vi "Teleop.vi"(10 "Match Info":T1={"Autonomous Elapsed Seconds"=0.0, "TeleOp Elapsed Seconds"=0.0, "Disabled Elapsed Seconds"=0.0, "Visited Autonomous"=FALSE, "Visited TeleOp"=FALSE, "Visited Disabled"=FALSE, "Autonomous Settings"={"Autonomous Style"=enum."Independent", "VI Refnum"=refnum}}, 11 "Call Context":T2) -> ()   [LabVIEW 2018]
doc: "This VI is called for each TeleOp packet received from the DS where the robot is not disabled. It is often used to read from the joysticks and update I/O or to update setpoints for timed control loops. It should complete and return within 20 milliseconds or it may miss DS packets."
uses:
  <vilib>/Rock Robotics/WPI/DriverStation/WPI_DriverStationDerivedRobotMode.ctl
  <vilib>/Rock Robotics/WPI/DriverStation/WPI_DriverStationMatch Info.ctl
  <vilib>/Rock Robotics/WPI/ThirdParty/Phoenix-LabVIEW/Motor Controller/Controls/CTRE_Phoenix_MotorControl_ControlMode.ctl
  <vilib>/Rock Robotics/Network Tables/NT Read Boolean.vi
  <vilib>/Rock Robotics/Network Tables/NT Read Number.vi
  <vilib>/Rock Robotics/WPI/Utilities/WPI_GetSetVariantRefNum.vi
  <vilib>/Rock Robotics/Network Tables/NT Write Boolean Array.vi
  <vilib>/Rock Robotics/Network Tables/NT Write Numeric Array.vi
  <vilib>/Rock Robotics/WPI/ThirdParty/Phoenix-LabVIEW/Motor Controller/Get/CTRE_Phoenix_MotorController_GetSelectedSensorData.vi
panel:
  out "Angle Back Left":dbl
  out "Angle Back Right":dbl
  out "Angle Front Right":dbl
  out "Angle Front Left":dbl
  out "Speed Back Left":dbl
  out "Speed Back Right":dbl
  out "Speed Front Right":dbl
  out "Speed Front Left":dbl
  in  "reverse steer":bool=TRUE
  in  "reverse encoder":bool=TRUE
  in  "ScaleSpeed":dbl=1.0
  in  "upper limit":dbl=0.02
  in  "lower limit":dbl=-0.02
  in  "Wheelbase":dbl=23.75
  in  "Trackwidth":dbl=18.1
  out "Sample Slider 0":dbl(slide) scale=0.0..5.0
  out "Sample Boolean 1":bool
  out "Sample Boolean 0":bool
  # "This column has configuration\nconstants for the swerve\ndrives. ReverseSteer and \nRevereEncoder should stay\n\"on\" (true) unless your hardware\nrequires it to be set otherwise."
  # "This column is debug \noutput for the 4 swerve\ndrives - wheel speed and \nangle info."
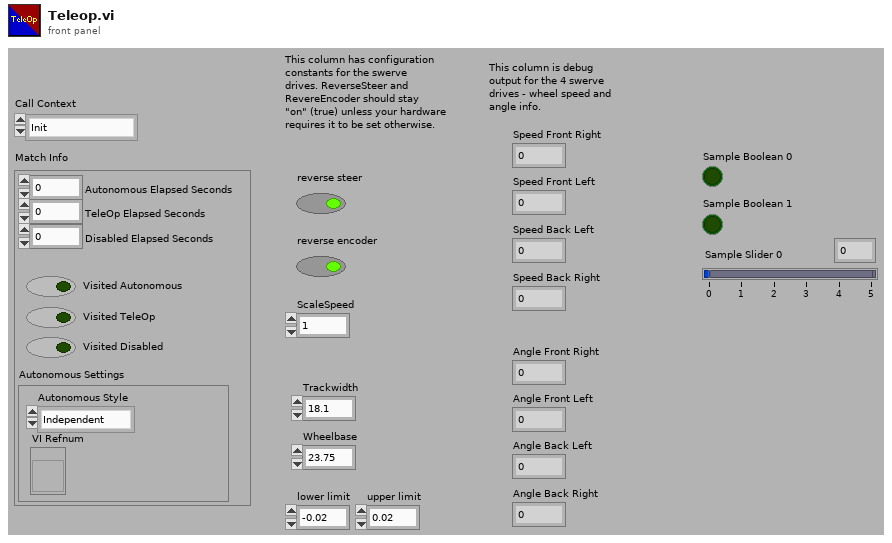
[diagram p1: front panel]
types:
  T1 = typedef "WPI_DriverStationMatch Info.ctl" = cluster{"Autonomous Elapsed Seconds":dbl, "TeleOp Elapsed Seconds":dbl, "Disabled Elapsed Seconds":dbl, "Visited Autonomous":bool, "Visited TeleOp":bool, "Visited Disabled":bool, "Autonomous Settings":cluster{"Autonomous Style":enum16{"Iterative", "Independent"}, "VI Refnum":refnum<vi>}}
  T2 = typedef "WPI_DriverStationDerivedRobotMode.ctl" = enum16{"Init", "Execute", "Stop"}
  T3 = typedef "CTRE_Phoenix_MotorControl_ControlMode.ctl" = u16
  T4 = typedef "WPI_JoystickDevRef.ctl" = cluster{"Device":T5}
  T5 = typedef "WPI_JoystickDeviceEnum.ctl" = enum16{"USB 0", "USB 1", "USB 2", "USB 3", "USB 4", "USB 5"}
  T6 = typedef "WPI_MotorControlDeviceRef.ctl" = cluster{"DeviceStatus":errorcluster, "Type":T7, "PWM":cluster{"PWM Channel":T8, "DeadBand":T9}, "CAN":cluster{"Device Number":u8, "SetOutput VI Ref":variant, "GetOutput VI Ref":variant, "Enable VI Ref":variant, "Disable VI Ref":variant, "Data":variant}, "Invert":bool, "DIO PWM":cluster{"PWM \"Enable\" Channel":T8, "DIOChannel":T10, "PWM Rate":dbl}}
  T7 = typedef "WPI_MotorControlType.ctl" = enum16{"PWM", "CAN", "DIO PWM"}
  T8 = typedef "FPGA_DIOPWMChannel.ctl" = enum8{"PWM 0", "PWM 1", "PWM 2", "PWM 3", "PWM 4", "PWM 5", "PWM 6", "PWM 7", "PWM 8", "PWM 9", "PWM MXP 0", "PWM MXP 1", "PWM MXP 2", "PWM MXP 3", "PWM MXP 4", "PWM MXP 5", "PWM MXP 6", "PWM MXP 7", "PWM MXP 8", "PWM MXP 9", "Invalid"}
  T9 = typedef "WPI_PWMDeadband.ctl" = cluster{"Name":string, "maxPositivePwm":i32, "minPositivePwm":i32, "centerPwm":i32, "maxNegativePwm":i32, "minNegativePwm":i32, "angularRange":u16}
  T10 = typedef "FPGA_DIOChannel.ctl" = enum8{"DIO 0", "DIO 1", "DIO 2", "DIO 3", "DIO 4", "DIO 5", "DIO 6", "DIO 7", "DIO 8", "DIO 9", "DIO MXP 0", "DIO MXP 1", "DIO MXP 2", "DIO MXP 3", "DIO MXP 4", "DIO MXP 5", "DIO MXP 6", "DIO MXP 7", "DIO MXP 8", "DIO MXP 9", "DIO MXP 10", "DIO MXP 11", "DIO MXP 12", "DIO MXP 13", "DIO MXP 14", "DIO MXP 15", "SPI Port CS1", "SPI Port CS2", "SPI Port CS3", "SPI Port MISO", "SPI Port MOSI", "Invalid"}
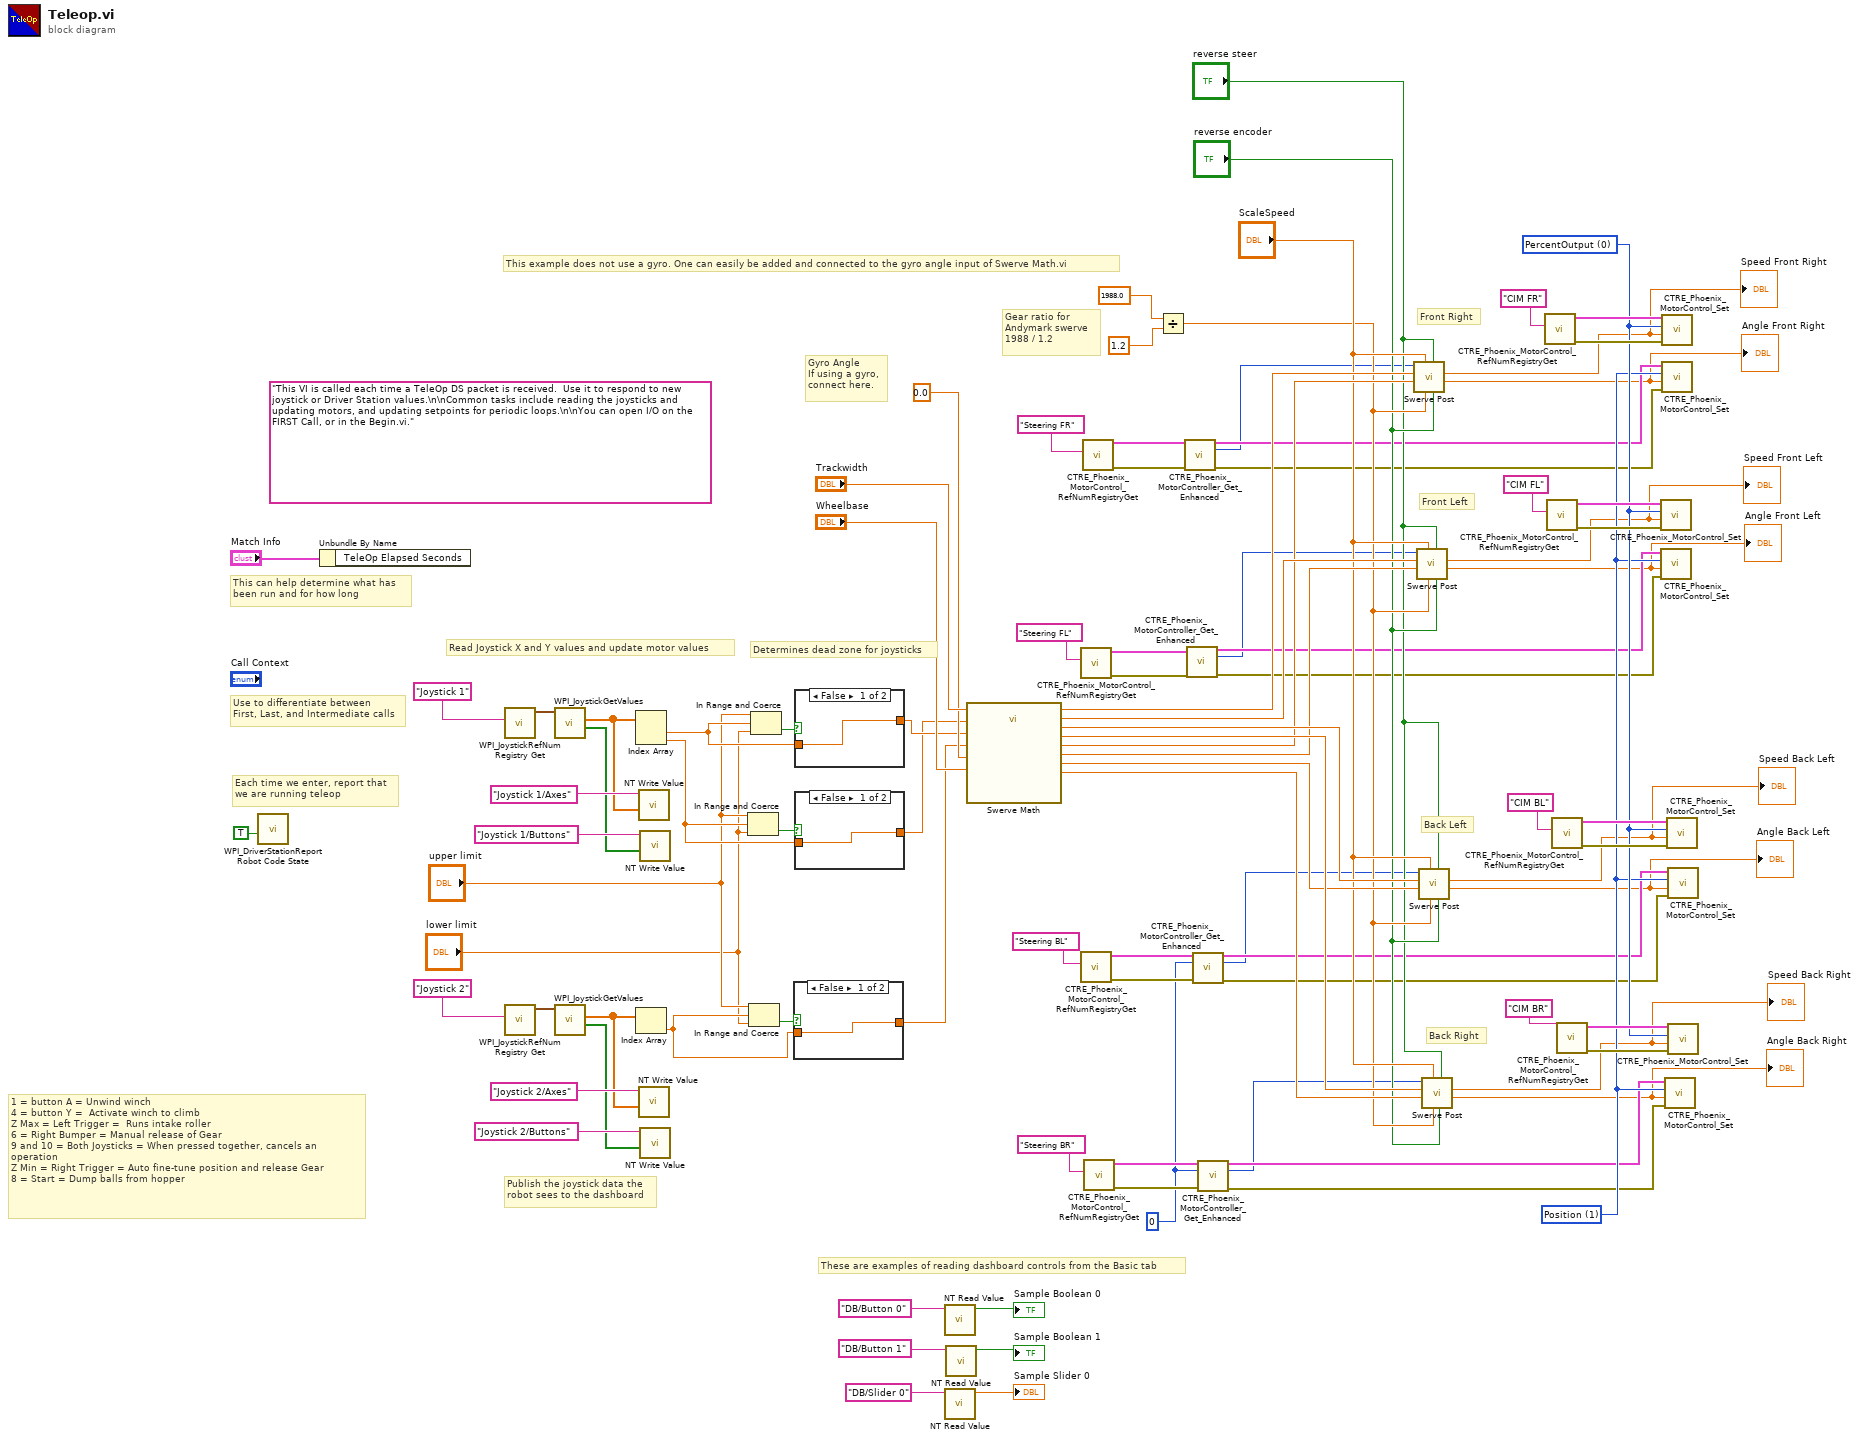
[diagram p0: block diagram]
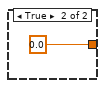
[diagram p2: hidden frame]
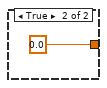
[diagram p3: hidden frame]
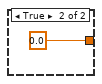
[diagram p4: hidden frame]
diagram:
  w22 = u32 0 ("pidLoopIdx")
  w31 = T3 1 items=["PercentOutput"=0, "Position"=1, "Velocity"=2, "Current"=3, "Follower"=5, "MotionProfile"=6, "MotionMagic"=7, "MotionProfileArc"=10, "Disabled"=15] ("Control Mode")
  w32 = T3 0 items=["PercentOutput"=0, "Position"=1, "Velocity"=2, "Current"=3, "Follower"=5, "MotionProfile"=6, "MotionMagic"=7, "MotionProfileArc"=10, "Disabled"=15] ("Control Mode")
  (unwired) "This VI is called each time a TeleOp DS packet is received.  Use it to respond to new joystick or Driver Station values.\n\nCommon tasks include reading the joysticks and updating motors, and updating setpoints for periodic loops.\n\nYou can open I/O on the FIRST Call, or in the Begin.vi."
  # "Gear ratio for\nAndymark swerve\n1988 / 1.2"
  # "Back Right"
  # "Back Left"
  # "Front Left"
  # "Front Right"
  # "This example does not use a gyro. One can easily be added and connected to the gyro angle input of Swerve Math.vi"
  # "1 = button A =\tUnwind winch\n4 = button Y = \tActivate winch to climb\nZ Max = Left Trigger = \tRuns intake roller\n6 = Right Bumper = Manual release of Gear\n9 and 10 = Both Joysticks = When pressed together, cancels an operation\nZ Min = Right Trigger = Auto fine-tune position and release Gear \n8 = Start = Dump balls from hopper"
  # "Determines dead zone for joysticks"
  # "Gyro Angle\nIf using a gyro,\nconnect here."
  # "Publish the joystick data the\nrobot sees to the dashboard"
  # "These are examples of reading dashboard controls from the Basic tab"
  # "Each time we enter, report that\nwe are running teleop"
  # "Use to differentiate between\nFirst, Last, and Intermediate calls"
  # "This can help determine what has\nbeen run and for how long"
  # "Read Joystick X and Y values and update motor values"
  n1 = call <vilib>:"WPI_DriverStationReport Robot Code State.vi"("TeleOp"=TRUE ("Autonomous")) -> ()  [unwired: 10 in, 1 out]
  n2 = Unbundle By Name("Match Info") -> ()  [unwired: 1 out]
  n3 = call <vilib>:"WPI_JoystickRefNum Registry Get.vi"("refnum name"="Joystick 1") -> ("JoystickDevRef"=w86:T4)  [unwired: 1 in, 9 out]
  n4 = call <vilib>:"WPI_JoystickRefNum Registry Get.vi"("refnum name"="Joystick 2") -> ("JoystickDevRef"=w80:T4)  [unwired: 1 in, 9 out]
  n5 = call <vilib>:"WPI_JoystickGetValues.vi"("JoystickDevRef"=w86) -> ("Buttons"=w82:bool[], "Axes"=w83:dbl[])  [unwired: 6 in, 3 out]
  n6 = call <vilib>:"WPI_JoystickGetValues.vi"("JoystickDevRef"=w80) -> ("Buttons"=w76:bool[], "Axes"=w77:dbl[])  [unwired: 6 in, 3 out]
  n7 = Index Array(array=w83) -> (element #1=w56:dbl, element #2=w58:dbl)  [unwired: 2 in]
  n8 = Index Array(array=w77) -> (element=w57:dbl)  [unwired: 1 in]
  n9 = call-poly <vilib>:"NT Write Value.vi"("Numeric Array"=w83, "Name"="Joystick 1/Axes") -> ()  [unwired: 9 in, 1 out]
  n10 = call-poly <vilib>:"NT Write Value.vi"("Numeric Array"=w77, "Name"="Joystick 2/Axes") -> ()  [unwired: 9 in, 1 out]
  n11 = call-poly <vilib>:"NT Write Value.vi"("Boolean Array"=w82, "Name"="Joystick 1/Buttons") -> ()  [unwired: 9 in, 1 out]
  n12 = call-poly <vilib>:"NT Write Value.vi"("Boolean Array"=w76, "Name"="Joystick 2/Buttons") -> ()  [unwired: 9 in, 1 out]
  n13 = In Range and Coerce(upper limit="upper limit", x=w58, lower limit="lower limit") -> (In Range?=w63:bool)  [unwired: 1 out]
  n14 = In Range and Coerce(upper limit="upper limit", x=w57, lower limit="lower limit") -> (In Range?=w64:bool)  [unwired: 1 out]
  n15 = In Range and Coerce(upper limit="upper limit", x=w56, lower limit="lower limit") -> (In Range?=w62:bool)  [unwired: 1 out]
  n16 = case shown="False" w64 {
    tunnel: [w96 0.0 ("Gyro Angle")] -> w61
    tunnel: w57 -> [w96 _]
    frame False {
    }
    frame True {
    }
  }
  n17 = case shown="False" w62 {
    tunnel: [w98 0.0 ("Gyro Angle")] -> w60
    tunnel: w56 -> [w98 _]
    frame False {
    }
    frame True {
    }
  }
  n18 = case shown="False" w63 {
    tunnel: [w100 0.0 ("Gyro Angle")] -> w59
    tunnel: w58 -> [w100 _]
    frame False {
    }
    frame True {
    }
  }
  n19 = call-poly <vilib>:"NT Read Value.vi"("Name"="DB/Button 0" ("refnum name")) -> ("Boolean"=→"Sample Boolean 0":bool)  [unwired: 9 in, 1 out]
  n20 = call-poly <vilib>:"NT Read Value.vi"("Name"="DB/Slider 0" ("refnum name")) -> ("Numeric"=→"Sample Slider 0":dbl)  [unwired: 9 in, 1 out]
  n21 = call-poly <vilib>:"NT Read Value.vi"("Name"="DB/Button 1" ("refnum name")) -> ("Boolean"=→"Sample Boolean 1":bool)  [unwired: 9 in, 1 out]
  n22 = call "Swerve Math.vi"("Trackwidth (W)"="Trackwidth", "Wheelbase (L)"="Wheelbase", "Y -FWD"=w59, "X1 STR"=w60, "X2 RCW"=w61, "Gyro Angle in degrees"=0.0 ("Gyro Angle")) -> ("wa3"=w47:dbl, "wa4"=w46:dbl, "ws1"=w52:dbl, "ws2"=w51:dbl, "ws3"=w50:dbl, "ws4"=w53:dbl, "wa2"=w48:dbl, "wa1"=w49:dbl)  [unwired: 2 in]
  n23 = call <vilib>:"CTRE_Phoenix_MotorControl_RefNumRegistryGet.vi"("refnum name"="Steering FL") -> ("error out"=w17:errorcluster, "PhoenixMotorControlDevRef"=w18:T6)  [unwired: 9 in]
  n24 = call <vilib>:"CTRE_Phoenix_MotorControl_RefNumRegistryGet.vi"("refnum name"="Steering BL") -> ("error out"=w26:errorcluster, "PhoenixMotorControlDevRef"=w27:T6)  [unwired: 9 in]
  n25 = call <vilib>:"CTRE_Phoenix_MotorControl_RefNumRegistryGet.vi"("refnum name"="Steering FR") -> ("error out"=w12:errorcluster, "PhoenixMotorControlDevRef"=w13:T6)  [unwired: 9 in]
  n26 = call <vilib>:"CTRE_Phoenix_MotorControl_RefNumRegistryGet.vi"("refnum name"="Steering BR") -> ("error out"=w28:errorcluster, "PhoenixMotorControlDevRef"=w29:T6)  [unwired: 9 in]
  n27 = Divide(x=1988.0, y=1.2) -> (x/y=w42:dbl)
  n28 = call-poly <vilib>:"CTRE_Phoenix_MotorController_Get_Enhanced.vi"("PhoenixMotorControlDevRef"=w13, "error in"=w12) -> ("PhoenixMotorControlDevRef"=w10:T6, "Position (Raw Sensor Units)"=w9:i32, "error out"=w11:errorcluster)  [unwired: 10 in, 1 out]
  n29 = call-poly <vilib>:"CTRE_Phoenix_MotorController_Get_Enhanced.vi"("PhoenixMotorControlDevRef"=w18, "error in"=w17) -> ("PhoenixMotorControlDevRef"=w15:T6, "Position (Raw Sensor Units)"=w14:i32, "error out"=w16:errorcluster)  [unwired: 10 in, 1 out]
  n30 = call-poly <vilib>:"CTRE_Phoenix_MotorController_Get_Enhanced.vi"("PhoenixMotorControlDevRef"=w27, "pidLoopIdx"=w22, "error in"=w26) -> ("PhoenixMotorControlDevRef"=w24:T6, "Position (Raw Sensor Units)"=w23:i32, "error out"=w25:errorcluster)  [unwired: 9 in, 1 out]
  n31 = call-poly <vilib>:"CTRE_Phoenix_MotorController_Get_Enhanced.vi"("PhoenixMotorControlDevRef"=w29, "pidLoopIdx"=w22, "error in"=w28) -> ("PhoenixMotorControlDevRef"=w20:T6, "Position (Raw Sensor Units)"=w19:i32, "error out"=w21:errorcluster)  [unwired: 9 in, 1 out]
  n32 = call "Swerve Post.vi"("reverse encoder"="reverse encoder", "reverse steer"="reverse steer", "gear ratio"=w42, "ScaleSpeed"="ScaleSpeed", "wa in"=w49, "ws in"=w52, "encoder in"=w9) -> ("wa out"=w2:dbl, "ws out 0-1"=w1:dbl)  [unwired: 3 in]
  "Speed Front Right" <- w1
  "Angle Front Right" <- w2
  n33 = call "Swerve Post.vi"("reverse encoder"="reverse encoder", "reverse steer"="reverse steer", "gear ratio"=w42, "ScaleSpeed"="ScaleSpeed", "wa in"=w48, "ws in"=w51, "encoder in"=w14) -> ("wa out"=w4:dbl, "ws out 0-1"=w3:dbl)  [unwired: 3 in]
  "Speed Front Left" <- w3
  "Angle Front Left" <- w4
  n34 = call "Swerve Post.vi"("reverse encoder"="reverse encoder", "reverse steer"="reverse steer", "gear ratio"=w42, "ScaleSpeed"="ScaleSpeed", "wa in"=w47, "ws in"=w50, "encoder in"=w23) -> ("wa out"=w6:dbl, "ws out 0-1"=w5:dbl)  [unwired: 3 in]
  "Speed Back Left" <- w5
  "Angle Back Left" <- w6
  n35 = call "Swerve Post.vi"("reverse encoder"="reverse encoder", "reverse steer"="reverse steer", "gear ratio"=w42, "ScaleSpeed"="ScaleSpeed", "wa in"=w46, "ws in"=w53, "encoder in"=w19) -> ("wa out"=w8:dbl, "ws out 0-1"=w7:dbl)  [unwired: 3 in]
  "Speed Back Right" <- w7
  "Angle Back Right" <- w8
  n36 = call <vilib>:"CTRE_Phoenix_MotorControl_RefNumRegistryGet.vi"("refnum name"="CIM FR") -> ("error out"=w39:errorcluster, "PhoenixMotorControlDevRef"=w40:T6)  [unwired: 9 in]
  n37 = call <vilib>:"CTRE_Phoenix_MotorControl_RefNumRegistryGet.vi"("refnum name"="CIM FL") -> ("error out"=w37:errorcluster, "PhoenixMotorControlDevRef"=w38:T6)  [unwired: 9 in]
  n38 = call <vilib>:"CTRE_Phoenix_MotorControl_RefNumRegistryGet.vi"("refnum name"="CIM BL") -> ("error out"=w35:errorcluster, "PhoenixMotorControlDevRef"=w36:T6)  [unwired: 9 in]
  n39 = call <vilib>:"CTRE_Phoenix_MotorControl_RefNumRegistryGet.vi"("refnum name"="CIM BR") -> ("error out"=w33:errorcluster, "PhoenixMotorControlDevRef"=w34:T6)  [unwired: 9 in]
  n40 = call <vilib>:"CTRE_Phoenix_MotorControl_Set.vi"("error in (no error)"=w37, "Output"=w3, "Control Mode"=w32, "PhoenixMotorControlDevRef"=w38) -> ()  [unwired: 6 in, 2 out]
  n41 = call <vilib>:"CTRE_Phoenix_MotorControl_Set.vi"("error in (no error)"=w16, "Output"=w4, "Control Mode"=w31, "PhoenixMotorControlDevRef"=w15) -> ()  [unwired: 6 in, 2 out]
  n42 = call <vilib>:"CTRE_Phoenix_MotorControl_Set.vi"("error in (no error)"=w39, "Output"=w1, "Control Mode"=w32, "PhoenixMotorControlDevRef"=w40) -> ()  [unwired: 6 in, 2 out]
  n43 = call <vilib>:"CTRE_Phoenix_MotorControl_Set.vi"("error in (no error)"=w11, "Output"=w2, "Control Mode"=w31, "PhoenixMotorControlDevRef"=w10) -> ()  [unwired: 6 in, 2 out]
  n44 = call <vilib>:"CTRE_Phoenix_MotorControl_Set.vi"("error in (no error)"=w21, "Output"=w8, "Control Mode"=w31, "PhoenixMotorControlDevRef"=w20) -> ()  [unwired: 6 in, 2 out]
  n45 = call <vilib>:"CTRE_Phoenix_MotorControl_Set.vi"("error in (no error)"=w35, "Output"=w5, "Control Mode"=w32, "PhoenixMotorControlDevRef"=w36) -> ()  [unwired: 6 in, 2 out]
  n46 = call <vilib>:"CTRE_Phoenix_MotorControl_Set.vi"("error in (no error)"=w25, "Output"=w6, "Control Mode"=w31, "PhoenixMotorControlDevRef"=w24) -> ()  [unwired: 6 in, 2 out]
  n47 = call <vilib>:"CTRE_Phoenix_MotorControl_Set.vi"("error in (no error)"=w33, "Output"=w7, "Control Mode"=w32, "PhoenixMotorControlDevRef"=w34) -> ()  [unwired: 6 in, 2 out]
